vi "ACQ Start.vi"(8 "error in (no error)":errorcluster, 11 "Conection Data":T1={"VISA resource name"="COM4"}) -> (0 "error out":errorcluster, 3 "Conection Data Out":T1={"VISA resource name"="COM4"})   [LabVIEW 2014, in "SJ-210 Lib.lvlib"]
doc: "Inicia el proceso de adquisición de datos del Rugosimetro."
uses:
  SJ-210 Lib.lvlib
  Typedef/Connection Data.ctl
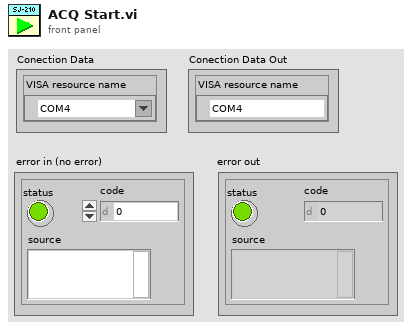
[diagram p1: front panel]
types:
  T1 = typedef "SJ-210 Lib.lvlib/Connection Data.ctl" = cluster{"VISA resource name":refnum<visa-resource-name>}
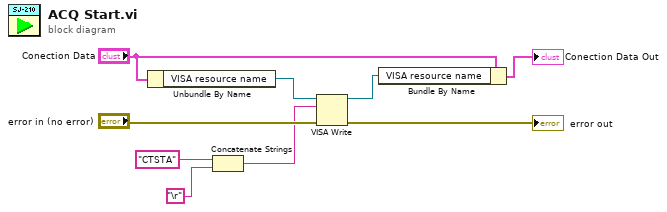
[diagram p0: block diagram]
diagram:
  n1 = Unbundle By Name("Conection Data") -> ("VISA resource name"=w8:refnum<visa-resource-name>)
  n2 = Concatenate Strings("CTSTA" ("write buffer"), "\r") -> (w5:string)
  n3 = VISA Write(VISA resource name=w8, write buffer=w5, error in (no error)="error in (no error)") -> (VISA resource name out=w2:refnum<visa-resource-name>, error out=→"error out":errorcluster)  [unwired: 1 out]
  n4 = Bundle By Name(cluster="Conection Data", "VISA resource name"=w2) -> (→"Conection Data Out":T1)
